vi "Init.vi"(4 "Message Cfg":T1={"EnTermChar"=TRUE, "termChar"=10, "suppEnEnRd"=TRUE, "sendEndEn"=FALSE} {"termChar" format="%.0x"}, 6 "timeout":u32=1000, 7 "Name":string="CPC_3010", 8 "error in":errorcluster, 9 "serialCfg":T2={"baud rate (9600)"=9600, "data bits (8)"=7, "stop bits (10: 1 bit)"=10, "parity (0:none)"=enum."Even", "flow control (0:none)"=0, "endModeforReads"=0, "endModeforWrites"=0} {"endModeforWrites" items=["None", "Last Bit", "TermChar", "Break"]; "endModeforReads" items=["None", "Last Bit", "TermChar"]; "flow control (0:none)" items=["None", "XON/XOFF", "RTS/CTS", "XON/XOFF & RTS/CTS", "DTR/DSR", "XON/XOFF & DTR/DSR"]; "stop bits (10: 1 bit)" items=["1.0"=10, "1.5"=15, "2.0"=20]; "data bits (8)" min=5 max=8 step=1}, 10 "Port":refnum<visa-resource-name>, 11 "3010 in":refnum<class "3010.lvclass">) -> (0 "error out":errorcluster, 3 "3010 out":refnum<class "3010.lvclass">)   [LabVIEW 2012, in "3010.lvclass"]
doc: "Initialize the TSI 3010 CPC. Set the termination character to a return character (0xD) for both the reads and writes. The baud rate should be 9600 and the communication should be set up for 7-e-1. These are the default so the only thing that the caller should have to do is set up the COM port."
uses:
  3010.lvclass
  <vilib>/Instr/_visa.llb/VISA Set IO Buffer Mask.ctl
  CPC.lvclass
  Reusable/Serial IO/Serial IO.lvclass
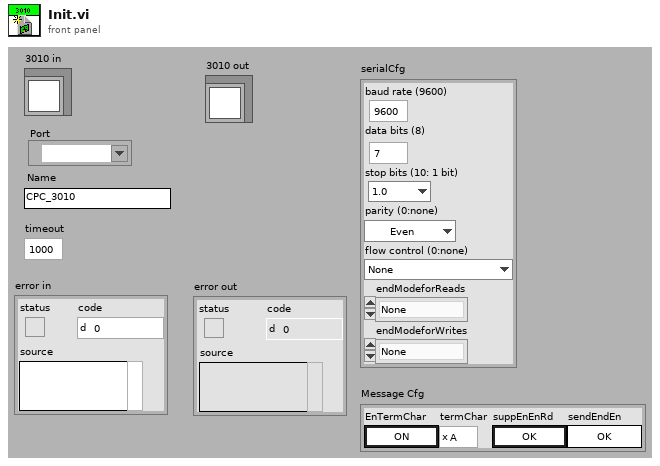
[diagram p1: front panel]
types:
  T1 = cluster{"EnTermChar":bool, "termChar":u8, "suppEnEnRd":bool, "sendEndEn":bool}
  T2 = cluster{"baud rate (9600)":u32, "data bits (8)":u16, "stop bits (10: 1 bit)":u16, "parity (0:none)":enum16{"None", "Odd", "Even", "Mark", "Space"}, "flow control (0:none)":u16, "endModeforReads":u16, "endModeforWrites":u16}
  T3 = typedef "VISA Set IO Buffer Mask.ctl" = u16
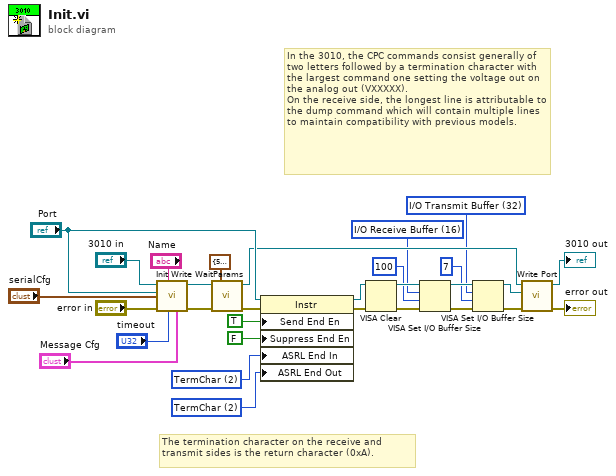
[diagram p0: block diagram]
diagram:
  w7 = T3 32 items=["I/O Receive Buffer"=16, "I/O Transmit Buffer"=32, "I/O Receive and Transmit Buffer"=48] ("Mask")
  w11 = T3 16 items=["I/O Receive Buffer"=16, "I/O Transmit Buffer"=32, "I/O Receive and Transmit Buffer"=48] ("Mask")
  w21 = u16 2 items=["None", "Last Bit", "TermChar", "Break"] ("Serial Settings:End Mode for Writes")
  w22 = u16 2 items=["None", "Last Bit", "TermChar"] ("Serial Settings:End Mode for Reads")
  # "The termination character on the receive and transmit sides is the return character (0xA)."
  # "In the 3010, the CPC commands consist generally of two letters followed by a termination character with the largest command one setting the voltage out on the analog out (VXXXXX).\nOn the receive side, the longest line is attributable to the dump command which will contain multiple lines to maintain compatibility with previous models."
  n1 = call-parent "Init.vi"("Message Cfg"="Message Cfg", "timeout"="timeout", "Name"="Name", "error in"="error in", "serialCfg"="serialCfg", "Port"="Port", "CPC in"="3010 in") -> ("error out"=w17:errorcluster, "CPC out"=w18:refnum<class "3010.lvclass">)  [unwired: 3 in]
  n2 = call "Write WaitParams.vi"("error in"=w17, "WaitParams"=cluster{"Timeout (ms)":u32, "LoopTime (ms)":u32} {"Timeout (ms)"=500, "LoopTime (ms)"=10}, "Serial IO in"=w18) -> ("error out"=w16:errorcluster, "Serial IO out"=w15:refnum<class "3010.lvclass">)  [unwired: 7 in]
  n3 = property class="Instr"(reference="Port", error in=w16, "Send End En"=TRUE ("Message Based Settings:Send End Enable"), "Suppress End En"=FALSE ("Message Based Settings:Suppress End Enable"), "ASRL End In"=w22, "ASRL End Out"=w21) -> (reference out=w19:refnum<visa-resource-name>, error out=w20:errorcluster)
  n4 = VISA Clear(VISA resource name=w19, error in (no error)=w20) -> (VISA resource name out=w13:refnum<visa-resource-name>, error out=w12:errorcluster)
  n5 = VISA Set I/O Buffer Size(VISA resource name=w13, mask (16)=w11, size (4096)=u32 100, error in (no error)=w12) -> (VISA resource name out=w8:refnum<visa-resource-name>, error out=w9:errorcluster)
  n6 = VISA Set I/O Buffer Size(VISA resource name=w8, mask (16)=w7, size (4096)=u32 7, error in (no error)=w9) -> (VISA resource name out=w5:refnum<visa-resource-name>, error out=w4:errorcluster)
  n7 = call-dynamic "Write Port.vi"("error in (no error)"=w4, "Port"=w5, "Serial IO in"=w15) -> ("error out"=→"error out":errorcluster, "Serial IO out"=→"3010 out":refnum<class "3010.lvclass">)  [unwired: 7 in]
